vi "Collide.vi"(8 "error in (no error)":errorcluster, 10 "ColliderObjects in":refnum<class "GameObject.lvclass">[](array[class]), 11 "Object in":refnum<class "GameObject.lvclass">) -> (0 "error out":errorcluster, 1 "collided":bool, 2 "ColliderObjects out":refnum<class "GameObject.lvclass">[](array[class]), 3 "Object out":refnum<class "GameObject.lvclass">)   [LabVIEW 2019, in "RT_Game.lvlib" / "GameObject.lvclass"]
uses:
  GameObject.lvclass
  GameObject.lvclass/GameObject.ctl
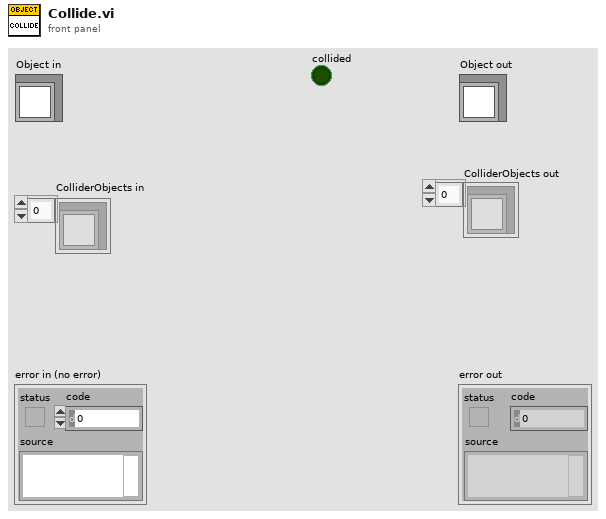
[diagram p1: front panel]
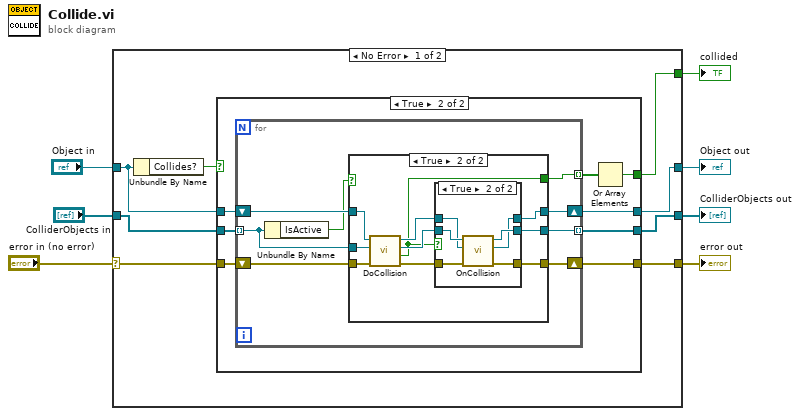
[diagram p0: block diagram]
diagram:
  n1 = case shown="No Error" "error in (no error)" {
    selector: "error in (no error)" -> [w15 w59]
    tunnel: [w13 w59] -> w6
    tunnel: [w12 w58] -> w5
    tunnel: "Object in" -> [w11 w58]
    tunnel: "ColliderObjects in" -> [w14 w57]
    tunnel: [w9 _] -> w2
    tunnel: [w8 w57] -> w1
    frame No Error {
      n2 = Unbundle By Name(w11) -> ("Collides?"=w10:bool)
      n3 = case shown="True" w10 {
        tunnel: w15 -> [w17 w26]
        tunnel: w11 -> [w18 w24]
        tunnel: w14 -> [w16 w23]
        tunnel: [w17 w25] -> w13
        tunnel: [w18 w22] -> w12
        tunnel: [_ w19] -> w9
        tunnel: [w16 w20] -> w8
        frame False {
        }
        frame True {
          n4 = for {
            shift-right: [w32] -> w25
            shift-left: w26 -> [w34]
            shift-right: [w30] -> w22
            shift-left: w24 -> [w29]
            tunnel: w23 -> [w28] mode=indexing
            tunnel: [w33] -> w21 mode=indexing
            tunnel: [w31] -> w20 mode=indexing
            n5 = Unbundle By Name(w28) -> ("IsActive"=w27:bool)
            n6 = case shown="True" w27 {
              tunnel: w34 -> [w37 w47]
              tunnel: [_ w38] -> w33
              tunnel: [w37 w45] -> w32
              tunnel: [w36 w44] -> w31
              tunnel: [w35 w43] -> w30
              tunnel: w28 -> [w36 w42]
              tunnel: w29 -> [w35 w41]
              frame False {
              }
              frame True {
                n7 = call "DoCollision.vi"("error in (no error)"=w47, "GameObject in"=w42, "Object in"=w41) -> ("error out"=w46:errorcluster, "Collided?"=w38:bool, "GameObject out"=w40:refnum<class "GameObject.lvclass">, "Object out"=w39:refnum<class "GameObject.lvclass">)  [unwired: 5 in]
                n8 = case shown="True" w38 {
                  tunnel: w46 -> [w48 w56]
                  tunnel: [w48 w55] -> w45
                  tunnel: [w50 w54] -> w44
                  tunnel: [w49 w53] -> w43
                  tunnel: w40 -> [w50 w52]
                  tunnel: w39 -> [w49 w51]
                  frame False {
                  }
                  frame True {
                    n9 = call-dynamic "OnCollision.vi"("error in (no error)"=w56, "Collider"=w51, "GameObject in"=w52) -> ("error out"=w55:errorcluster, "Colliderout"=w53:refnum<class "GameObject.lvclass">, "GameObject out"=w54:refnum<class "GameObject.lvclass">)  [unwired: 6 in]
                  }
                }
              }
            }
          }
          n10 = Or Array Elements(Boolean array=w21) -> (logical OR=w19:bool)
        }
      }
    }
    frame Error {
    }
  }
  "error out" <- w6
  "Object out" <- w5
  "collided" <- w2
  "ColliderObjects out" <- w1
